vi "SP Read Single.vi"(8 "error in":errorcluster, 9 "Channel Index":i32=1, 11 "Pressure Setpoint in":refnum<class "Pressure Setpoint.lvclass">) -> (0 "error out":errorcluster, 1 "Changed or First Call?":bool, 2 "Pressure SP":dbl, 3 "Pressure Setpoint out":refnum<class "Pressure Setpoint.lvclass">)   [LabVIEW 2023, in "Pressure Setpoint.lvclass"]
uses:
  Pressure Setpoint.lvclass
  Parents/Setpoint/Setpoint.lvclass
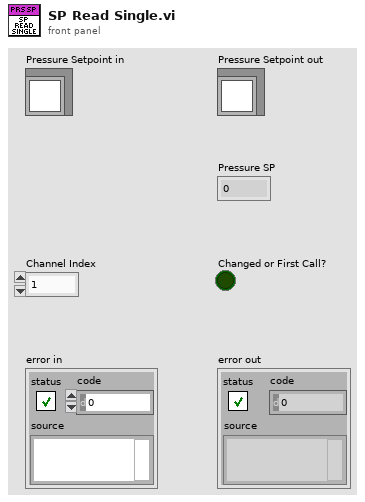
[diagram p1: front panel]
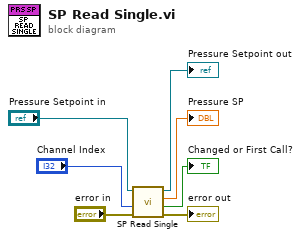
[diagram p0: block diagram]
diagram:
  n1 = call-parent "SP Read Single.vi"("error in"="error in", "Channel Index"="Channel Index", "Setpoint in"="Pressure Setpoint in") -> ("error out"=→"error out":errorcluster, "Changed or First Call?"=→"Changed or First Call?":bool, "Current SP"=→"Pressure SP":dbl, "Setpoint out"=→"Pressure Setpoint out":refnum<class "Pressure Setpoint.lvclass">)  [unwired: 5 in]
